vi "SR830.vi"(0 "GPIB address":string) -> (1 "x channel":dbl format="%.2e", 2 "y channel":dbl format="%.2e")   [LabVIEW 2013]
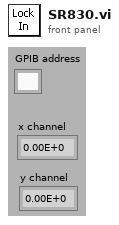
[diagram p1: front panel]
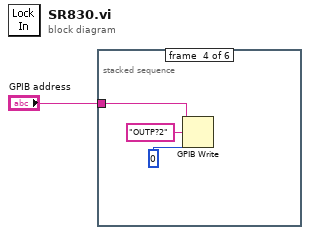
[diagram p0: block diagram]
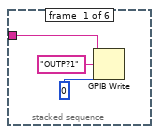
[diagram p2: hidden frame]
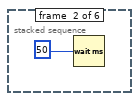
[diagram p3: hidden frame]
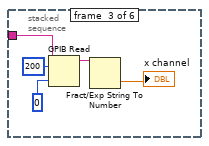
[diagram p4: hidden frame]
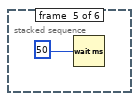
[diagram p5: hidden frame]
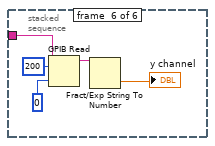
[diagram p6: hidden frame]
diagram:
  n1 = stacked-sequence {
    tunnel: "GPIB address" -> [w4 _ w10 w13 _ w19]
    frame #0 {
      n2 = GPIB Write(0:w4, 1:"OUTP?1", 2:0) -> ()  [unwired: 2 in, 2 out]
    }
    frame #1 {
      n3 = Wait (ms)(milliseconds to wait=50) -> ()  [unwired: 1 out]
    }
    frame #2 {
      n4 = GPIB Read(0:w10, 1:200, 2:0) -> (5:w9:string)  [unwired: 2 in, 2 out]
      n5 = Fract/Exp String To Number(string=w9) -> (number=→"x channel":dbl)  [unwired: 3 in, 1 out]
    }
    frame #3 {
      n6 = GPIB Write(0:w13, 1:"OUTP?2", 2:0) -> ()  [unwired: 2 in, 2 out]
    }
    frame #4 {
      n7 = Wait (ms)(milliseconds to wait=50) -> ()  [unwired: 1 out]
    }
    frame #5 {
      n8 = GPIB Read(0:w19, 1:200, 2:0) -> (5:w18:string)  [unwired: 2 in, 2 out]
      n9 = Fract/Exp String To Number(string=w18) -> (number=→"y channel":dbl)  [unwired: 3 in, 1 out]
    }
  }
